vi "ma_Inverse f Settings Check.vi"(8 "error in (no error)":errorcluster, 9 "filter specifications":T1={"lower cutoff freq"=0.1, "higher cutoff freq"=100.0, "order"=5} {"higher cutoff freq" format="%#_2p"; "lower cutoff freq" format="%#_2p"}, 10 "exponent":dbl=1.0 format="%.2g", 11 "sampling info":cluster{"Fs":dbl, "#s":dbl}={"Fs"=1000.0, "#s"=1000.0} {"Fs" format="%.2p"}) -> (0 "error out":errorcluster)   [LabVIEW 2020, in "NI_MABase.lvlib"]
doc: "Checks to make sure that each inverse f filter design parameter is within a valid range."
uses:
  NI_MABase.lvlib
  NI_AALBase.lvlib
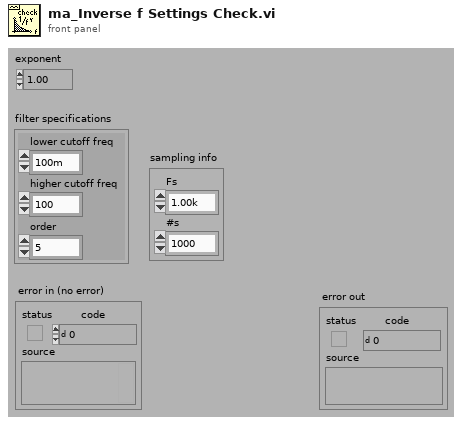
[diagram p1: front panel]
types:
  T1 = cluster{"lower cutoff freq":dbl, "higher cutoff freq":dbl, "order":i32}
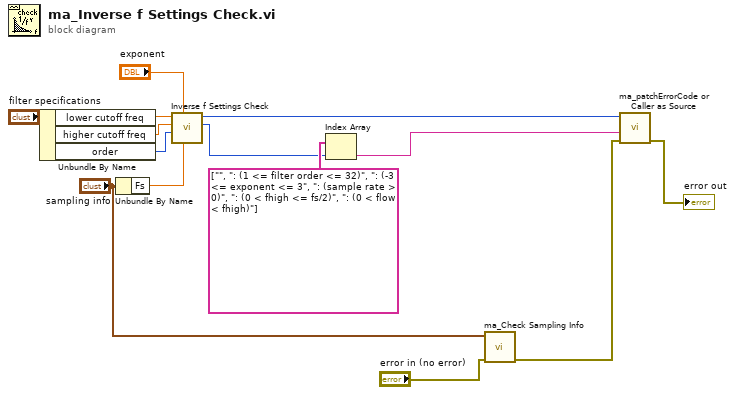
[diagram p0: block diagram]
diagram:
  n1 = Unbundle By Name("filter specifications") -> ("lower cutoff freq"=w6:dbl, "higher cutoff freq"=w5:dbl, "order"=w4:i32)
  n2 = Unbundle By Name("sampling info") -> ("Fs"=w8:dbl)
  n3 = call "Inverse f Settings Check.vi"("fs"=w8, "exponent"="exponent", "order"=w4, "higher cutoff freq"=w5, "lower cutoff freq"=w6) -> ("error index"=w10:i32, "error code"=w9:i32)  [unwired: 5 in]
  n4 = Index Array(array=string[] ["", ": (1 <= filter order <= 32)", ": (-3 <= exponent <= 3", ": (sample rate > 0)", ": (0 < fhigh <= fs/2)", ": (0 < flow < fhigh)"], index=w10) -> (element=w13:string)
  n5 = call "ma_Check Sampling Info.vi"("error in (no error)"="error in (no error)", "sampling info"="sampling info") -> ("error out"=w1:errorcluster)  [unwired: 4 in, 1 out]
  n6 = call "ma_patchErrorCode or Caller as Source.vi"("error in (no error)"=w1, "string to append to source"=w13, "error code"=w9) -> ("error out"=→"error out":errorcluster)  [unwired: 8 in]
